vi "Parse Supported Objects.vi"(8 "error in":errorcluster, 11 "EDS in":refnum<class "EDS.lvclass">) -> (0 "error out":errorcluster, 3 "EDS out":refnum<class "EDS.lvclass">)   [LabVIEW 2024, in "EDS.lvlib" / "EDS.lvclass"]
uses:
  EDS.lvclass
  EDS.lvclass/EDS.ctl
  Mandatory Objects/Mandatory Objects.lvclass
  D:/git/EDS-File-Viewer/Core/Supported Objects/Supported Objects.lvclass
  Optional Objects/Optional Objects.lvclass
  Manufacturer Objects/Manufacturer Objects.lvclass
  TypeDefinitions/TypeDefinitions.lvclass
  Supported Objects/Supported Objects.lvclass
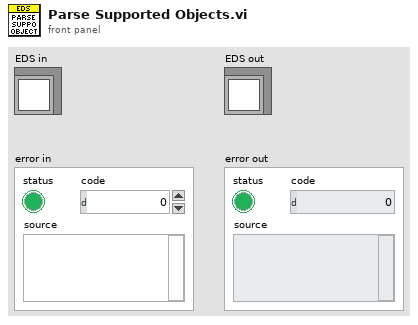
[diagram p1: front panel]
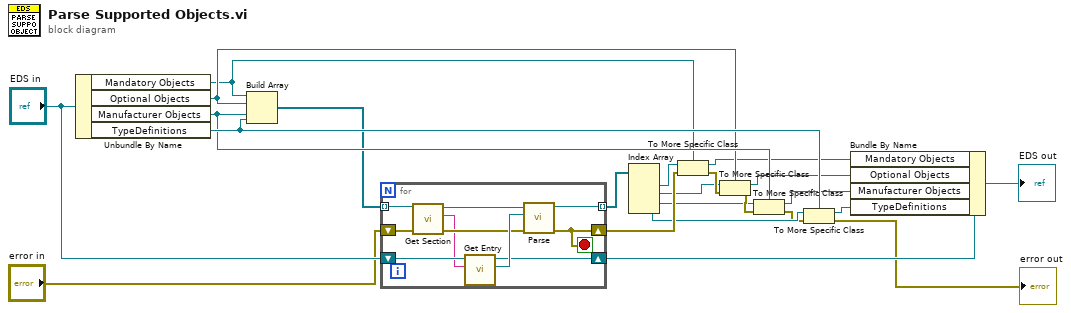
[diagram p0: block diagram]
diagram:
  n1 = Unbundle By Name("EDS in") -> ("Mandatory Objects"=w20:refnum<class "Mandatory Objects.lvclass">, "Optional Objects"=w21:refnum<class "Optional Objects.lvclass">, "Manufacturer Objects"=w22:refnum<class "Manufacturer Objects.lvclass">, "TypeDefinitions"=w23:refnum<class "TypeDefinitions.lvclass">)
  n2 = Build Array(w20, w21, w22, w23) -> (w4:refnum<class "Supported Objects.lvclass">[])
  n3 = for {
    tunnel: w4 -> [w26] mode=indexing
    shift-right: [w24] -> w17
    shift-left: "error in" -> [w30]
    tunnel: [w28] -> w5 mode=indexing
    shift-right: [w29] -> w19
    shift-left: "EDS in" -> [w32]
    stop <- w24 stop-if-true
    n4 = call-dynamic "Get Section.vi"("Supported Objects in"=w26) -> ("Section"=w27:string, "Supported Objects out"=w25:refnum<class "Supported Objects.lvclass">)  [unwired: 9 in]
    n5 = call "Get Entry.vi"("Section"=w27, "EDS in"=w32) -> ("Section"=w31:refnum<class "Section.lvclass">, "EDS out"=w29:refnum<class "EDS.lvclass">)  [unwired: 8 in]
    n6 = call-dynamic "Parse.vi"("error in"=w30, "Object Section"=w31, "Supported Objects in"=w25) -> ("error out"=w24:errorcluster, "Supported Objects out"=w28:refnum<class "Supported Objects.lvclass">)  [unwired: 7 in]
  }
  n7 = Index Array(array=w5) -> (element #1=w6:refnum<class "Supported Objects.lvclass">, element #2=w7:refnum<class "Supported Objects.lvclass">, element #3=w8:refnum<class "Supported Objects.lvclass">, element #4=w10:refnum<class "Supported Objects.lvclass">)  [unwired: 4 in]
  n8 = To More Specific Class(target class=w20, reference=w6, error in=w17) -> (specific class reference=w16:refnum<class "Mandatory Objects.lvclass">, error out=w11:errorcluster)
  n9 = To More Specific Class(target class=w21, reference=w7, error in=w11) -> (specific class reference=w15:refnum<class "Optional Objects.lvclass">, error out=w12:errorcluster)
  n10 = To More Specific Class(target class=w22, reference=w8, error in=w12) -> (specific class reference=w14:refnum<class "Manufacturer Objects.lvclass">, error out=w9:errorcluster)
  n11 = To More Specific Class(target class=w23, reference=w10, error in=w9) -> (specific class reference=w13:refnum<class "TypeDefinitions.lvclass">, error out=→"error out":errorcluster)
  n12 = Bundle By Name(cluster=w19, "Mandatory Objects"=w16, "Optional Objects"=w15, "Manufacturer Objects"=w14, "TypeDefinitions"=w13) -> (→"EDS out":refnum<class "EDS.lvclass">)
